vi "Read Lidar Data.vi"(8 "error in (no error)":errorcluster) -> (0 "error out":errorcluster, 2 "Direction":dbl[](array[numeric]), 3 "Magnitude":dbl[](array[numeric]))   [LabVIEW 2018]
uses:
  Lidar Globals.vi
  <instrlib>/Hokuyo URG Series/Hokuyo URG Series.lvlib
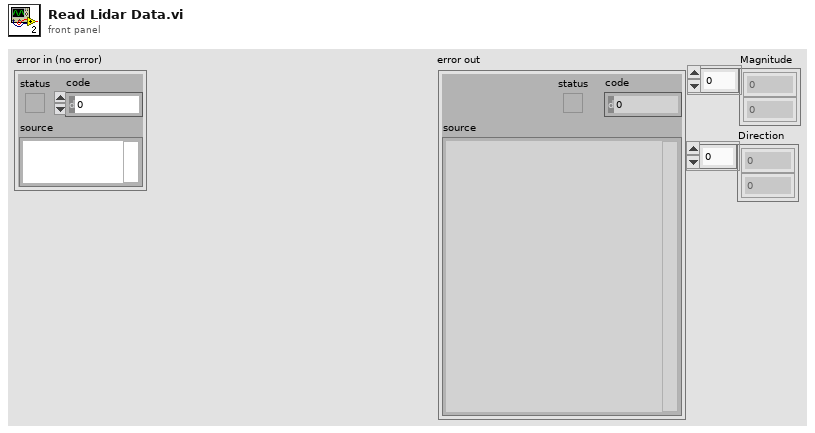
[diagram p1: front panel]
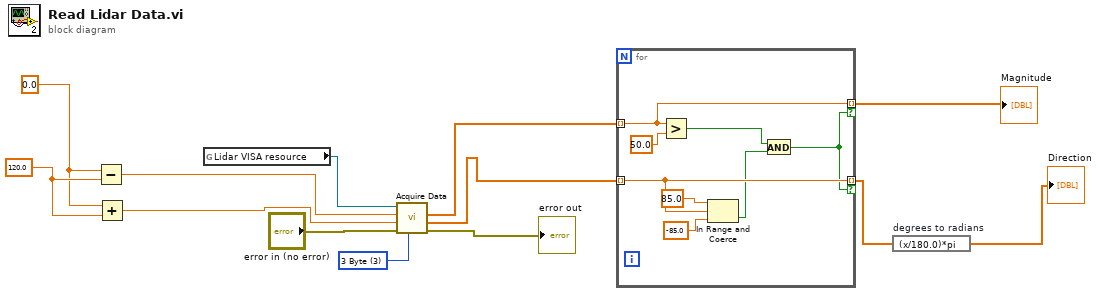
[diagram p0: block diagram]
diagram:
  w3 = u16 3 items=["2 Byte"=2, "3 Byte"=3] ("Data Encoding Width (3 Byte)")
  w10 = 120.0 ("y")
  w9 = 0.0 ("Start Point (-120°)")
  n1 = Subtract(x=w9, y=w10) -> (x-y=w7:dbl)
  n2 = Add(x=w9, y=w10) -> (x+y=w8:dbl)
  n3 = global read "Lidar Globals.vi" "Lidar VISA resource"() -> (w11:refnum<visa-resource-name>)
  n4 = call <instrlib>:"Acquire Data.vi"("Data Encoding Width (3 Byte)"=w3, "error in (no error)"="error in (no error)", "End Point (120°)"=w8, "Start Point (-120°)"=w7, "VISA resource name"=w11) -> ("error out"=→"error out":errorcluster, "Direction"=w4:dbl[], "Magnitude"=w6:dbl[])  [unwired: 3 in, 1 out]
  n5 = for {
    tunnel: w6 -> [w20] mode=indexing
    tunnel: w4 -> [w19] mode=indexing
    tunnel: [w20] -> w5 mode=indexing if=w14
    tunnel: [w19] -> w2 mode=indexing if=w14
    n6 = Greater?(x=w20, y=50.0) -> (0:w15:bool)
    n7 = In Range and Coerce(upper limit=85.0, x=w19, lower limit=-85.0 ("upper limit")) -> (In Range?=w16:bool)  [unwired: 1 out]
    n8 = And(x=w15, y=w16) -> (x .and. y?=w14:bool)
  }
  "Magnitude" <- w5
  n9 = expression code="(x/180.0)*pi" "degrees to radians"(w2) -> (→"Direction":dbl[])
